vi "Load Class on JSON Item Name.vi"(8 "error in (no error)":errorcluster, 10 "JSON Config":string, 11 "Abs_Type in":refnum<class "Abs_Type.lvclass">) -> (0 "error out":errorcluster, 3 "Abs_Type out":refnum<class "Abs_Type.lvclass">)   [LabVIEW 2021, in "Abs_Type.lvclass"]
uses:
  Abs_Type.lvclass
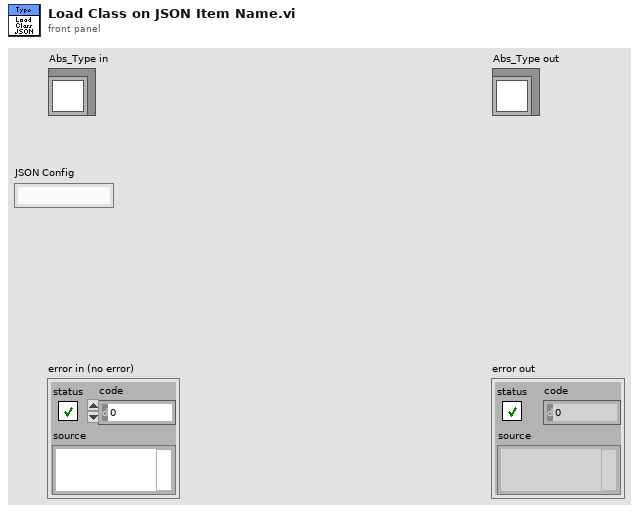
[diagram p1: front panel]
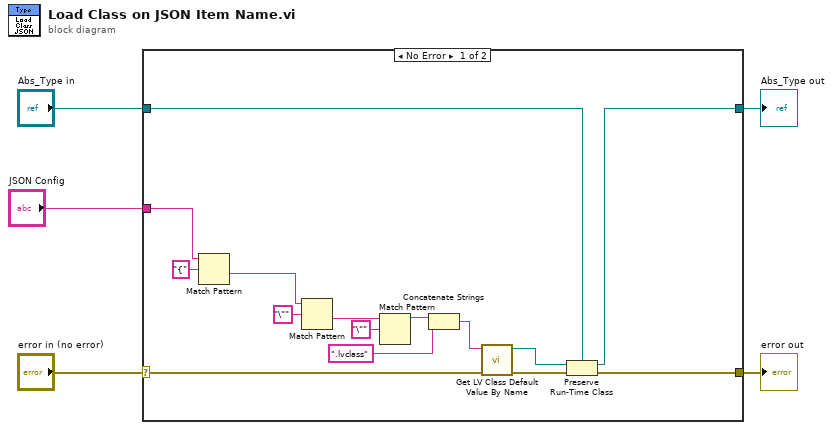
[diagram p0: block diagram]
diagram:
  n1 = case shown="No Error" "error in (no error)" {
    selector: "error in (no error)" -> [w12 w22]
    tunnel: [w9 w22] -> w4
    tunnel: [w10 w21] -> w2
    tunnel: "Abs_Type in" -> [w11 w21]
    tunnel: "JSON Config" -> [w7 _]
    frame No Error {
      n2 = Match Pattern(string=w7, regular expression="{") -> (after substring=w6:string)  [unwired: 1 in, 3 out]
      n3 = Match Pattern(string=w6, regular expression="\"") -> (after substring=w20:string)  [unwired: 1 in, 3 out]
      n4 = Match Pattern(string=w20, regular expression="\"") -> (before substring=w17:string)  [unwired: 1 in, 3 out]
      n5 = Concatenate Strings(w17, ".lvclass" ("string")) -> (w14:string)
      n6 = call <vilib>:"Get LV Class Default Value By Name.vi"("error in (no error)"=w12, "class name"=w14) -> ("error out"=w16:errorcluster, "object"=w15:refnum<class>)  [unwired: 8 in]
      n7 = Preserve Run-Time Class(object in=w15, error in=w16, 2:w11) -> (object out=w10:refnum<class "Abs_Type.lvclass">, error out=w9:errorcluster)
    }
    frame Error {
    }
  }
  "error out" <- w4
  "Abs_Type out" <- w2
